vi "ArgoBot_Close.vi"(11 "Write_Cluster":T7) -> ()   [LabVIEW 2018, in "ArgoBotLib.lvlib"]
uses:
  ArgoBotLib.lvlib
  <vilib>/MakerHub/LINX/Private/Type Defs/LINX Ref.ctl
  <vilib>/MakerHub/LINX/Private/Type Defs/Platform.ctl
  <vilib>/MakerHub/LINX/Private/Type Defs/Interface.ctl
  <vilib>/MakerHub/LINX/Private/Device/Type Defs/LINX Device Config.ctl
  <vilib>/MakerHub/LINX/Private/Device/Type Defs/TCP Config.ctl
  <vilib>/MakerHub/LINX/Private/Device/Type Defs/Channels.ctl
  <vilib>/Utility/inputDevices.llb/closeJoystick.vi
  <vilib>/MakerHub/LINX/Public/Sensors/Motion/Servo/Servo Close N Channels.vi
  <vilib>/MakerHub/LINX/LMH-LINX.lvlib
  <vilib>/MakerHub/LINX/Public/Sensors/Motion/Servo/Servo.lvlib
  <vilib>/MakerHub/LINX/Private/Device/Device.lvlib
panel:
  # "ArgoBot  Close"
  # "This vi close all connections"
  # "Inputs"
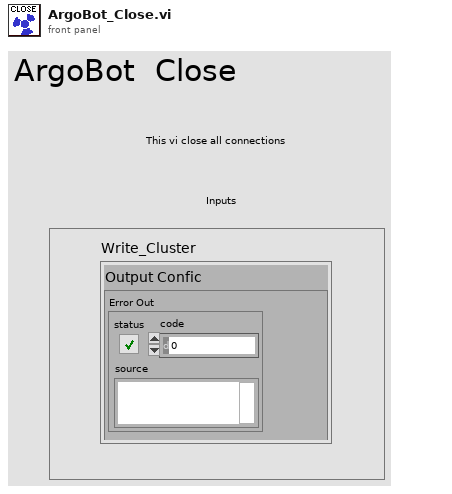
[diagram p1: front panel]
types:
  T1 = typedef "LMH-LINX.lvlib/LINX Ref.ctl" = cluster{"IO":T2, "Interface":T3, "LINX Device Config":T4}
  T2 = typedef "LMH-LINX.lvlib/Platform.ctl" = enum16{"Remote", "Local"}
  T3 = typedef "LMH-LINX.lvlib/Interface.ctl" = enum16{"Serial", "TCP"}
  T4 = typedef "LMH-LINX.lvlib/Device.lvlib/LINX Device Config.ctl" = cluster{"Interface":T3, "COM Port":refnum<visa-resource-name>, "TCP Configuration":T5, "Device Family":u8, "Device ID":u8, "Device Name":string, "TCP Ref":refnum<k5>, "Channels":T6}
  T5 = typedef "LMH-LINX.lvlib/Device.lvlib/TCP Config.ctl" = cluster{"IP Address":string, "Port":u16}
  T6 = typedef "LMH-LINX.lvlib/Channels.ctl" = cluster{"DI":u8[], "DO":u8[], "AI":u8[], "AO":u8[], "PWM":u8[], "QE":u8[], "UART":u8[], "I2C 2":u8[], "SPI":u8[], "CAN":u8[], "Servo":u8[], "AI Ref (V)":dbl, "AI Resolution (Bits)":u8, "AO Ref (V)":dbl, "AO Resolution (Bits)":u8}
  T7 = cluster{"Output Confic":cluster{"Error Out":errorcluster, "LINX Resource":T1}, "Joystick Read":cluster{"Joystick":cluster{"A":bool, "B":bool, "X":bool, " Y":bool, "Left_Trigger":dbl, "Right_Trigger ":dbl, "LB":bool, " RB":bool, "Left_Thumb_Button":bool, "Right_Thumb_Button":bool, "Stop_Back":bool, "Start":bool, "X_Axis_Left":dbl, "Y_Axis_Left":dbl, "X_Axis_Right":dbl, "Y_Axis_Right":dbl}, "Joystick error out":errorcluster, "Refnum out":refnum<k1>}, "Read Config":cluster{"Read_Config":i32[], "Error Out":errorcluster, "LINX Resource 2":T1}, "Read_Value":cluster{"Analog 1":dbl, "Analog 2":dbl, "Analog 3":dbl, "Voltage":dbl, "GPIO 1 Read":bool, "GPIO 2 Read":bool, "GPIO 3 Read":bool, "Loop Rate (Hz)":u32}, "Joystick error out":errorcluster, "Linx":cluster{"LINX Ref":T1, "Error Out":errorcluster}, "Setup":cluster{"Analog 1 Config":u16, "Analog 2 Config":u16, "Analog 3 Config":u16, "GPIO 1 Config":u16, "GPIO 2 Config":u16, "GPIO 3 Config":u16, "Drive Config":u16, "Motor Mode":u16, "Battery_Config":u16, "LED Config":u16}}
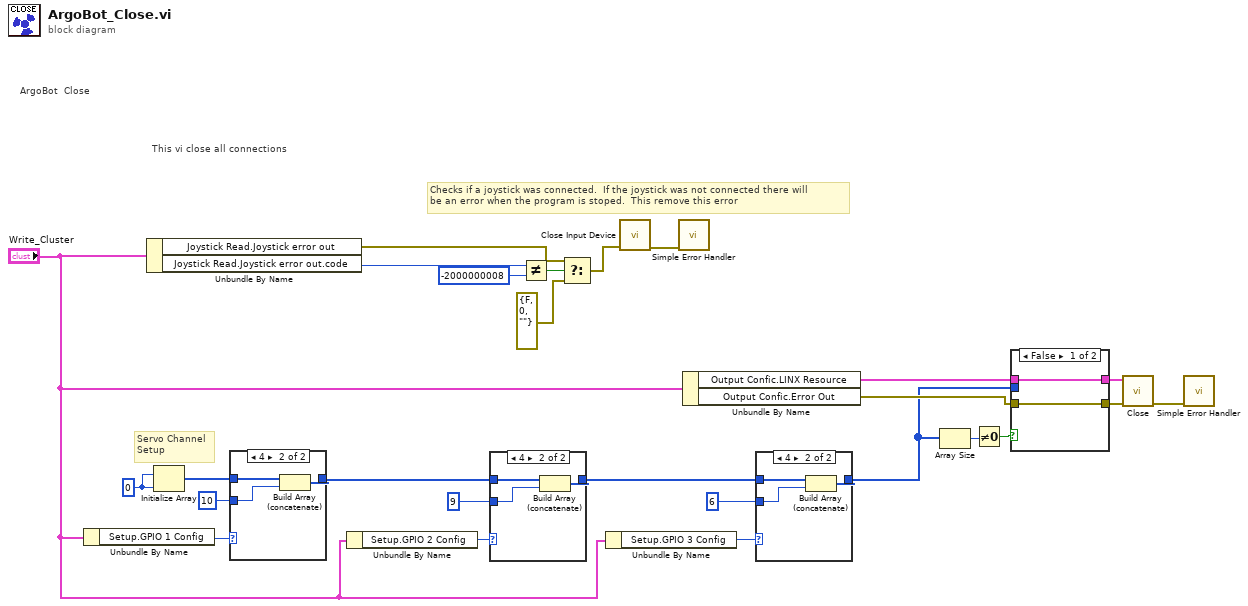
[diagram p0: block diagram]
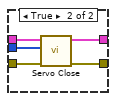
[diagram p2: hidden frame]
diagram:
  w20 = 0 ("dimension size")
  # "Servo Channel\nSetup"
  # "Checks if a joystick was connected.  If the joystick was not connected there will \nbe an error when the program is stoped.  This remove this error"
  # "This vi close all connections"
  # "ArgoBot  Close"
  n1 = Unbundle By Name("Write_Cluster") -> ("Setup.GPIO 1 Config"=w18:u16)
  n2 = Unbundle By Name("Write_Cluster") -> ("Joystick Read.Joystick error out"=w10:errorcluster, "Joystick Read.Joystick error out.code"=w9:i32)
  n3 = Initialize Array(w20, w20) -> (w19:i32[])
  n4 = case shown="4" w18 {
    tunnel: w19 -> [w27 w30]
    tunnel: [w27 w29] -> w14
    tunnel: 10 ("element") -> [_ w28]
    frame 0, Default {
    }
    frame 4 {
      n5 = Build Array (concatenate)(w30, w28) -> (w29:i32[])
    }
  }
  n6 = Unbundle By Name("Write_Cluster") -> ("Setup.GPIO 2 Config"=w15:u16)
  n7 = case shown="4" w15 {
    tunnel: w14 -> [w31 w34]
    tunnel: [w31 w33] -> w11
    tunnel: 9 ("element") -> [_ w32]
    frame 0, Default {
    }
    frame 4 {
      n8 = Build Array (concatenate)(w34, w32) -> (w33:i32[])
    }
  }
  n9 = Not Equal?(x=w9, y=-2000000008) -> (x != y?=w23:bool)
  n10 = Select(t=w10, s=w23, f=errorcluster {"status"=FALSE, "code"=0, "source"=""} ("error in (no error)")) -> (s? t:f=w21:errorcluster)
  n11 = Unbundle By Name("Write_Cluster") -> ("Setup.GPIO 3 Config"=w13:u16)
  n12 = call-poly <vilib>:"Close Input Device.vi"("error in (no error)"=w21) -> ("error out"=w26:errorcluster)  [unwired: 1 in, 8 out]
  n13 = call <vilib>:"Simple Error Handler.vi"("error in (no error)"=w26) -> ()  [unwired: 3 in, 6 out]
  n14 = Unbundle By Name("Write_Cluster") -> ("Output Confic.LINX Resource"=w7:T1, "Output Confic.Error Out"=w6:errorcluster)
  n15 = case shown="4" w13 {
    tunnel: w11 -> [w35 w38]
    tunnel: [w35 w37] -> w1
    tunnel: 6 ("element") -> [_ w36]
    frame 0, Default {
    }
    frame 4 {
      n16 = Build Array (concatenate)(w38, w36) -> (w37:i32[])
    }
  }
  n17 = Array Size(array=w1) -> (size(s)=w3:i32)
  n18 = Not Equal To 0?(x=w3) -> (x != 0?=w2:bool)
  n19 = case shown="False" w2 {
    tunnel: w7 -> [w40 w45]
    tunnel: w6 -> [w39 w44]
    tunnel: w1 -> [_ w43]
    tunnel: [w40 w42] -> w5
    tunnel: [w39 w41] -> w4
    frame False {
    }
    frame True {
      n20 = call-poly <vilib>:"Servo Close.vi"("Error In"=w44, "Servo Channels"=w43, "LINX Resource"=w45) -> ("Error Out"=w41:errorcluster, "LINX Resource"=w42:T1)  [unwired: 7 in]
    }
  }
  n21 = call <vilib>:"Close.vi"("Error In"=w4, "LINX Resource"=w5) -> ("Error Out"=w25:errorcluster)  [unwired: 9 in]
  n22 = call <vilib>:"Simple Error Handler.vi"("error in (no error)"=w25) -> ()  [unwired: 4 in, 5 out]
